vi "Add Alarm_Alarm.vi"(7 "SysDef Ref":T1, 8 "error in (no error)":errorcluster, 9 "Alarm Settings":T2={"Name"="", "Description"="", "Alarm Channel Node Path"="", "UpperLimit"=0.0, "Upper Limit Channel Node Path"="", "LowerLimit"=0.0, "Lower Limit Channel Node Path"="", "Alarm Action Node Path"="", "Mode"=0, "DefaultState"=1, "Priority"=0, "Delay"=0.0, "TripMessage"="", "GroupNumber"=0} {"Priority" items=["Low", "Medium", "High"]; "DefaultState" items=["Disabled", "Enabled"]; "Mode" items=["Normal", "IndicateOnly"]}, 11 "Alarm Folder Ref":refnum<k24>) -> (0 "error out":errorcluster, 3 "Alarm Folder Ref out":refnum<k24>)   [LabVIEW 2019, in "Simple SysDef API.lvlib"]
uses:
  <userlib>/SimpleSysDef/Simple SysDef API.lvlib
  NationalInstruments.VeriStand.SystemDefinitionAPI
  <userlib>/SimpleSysDef/_SubVIs/Add Alarm_Settings.ctl
  <userlib>/SimpleSysDef/_SubVIs/System Definition Reference.ctl
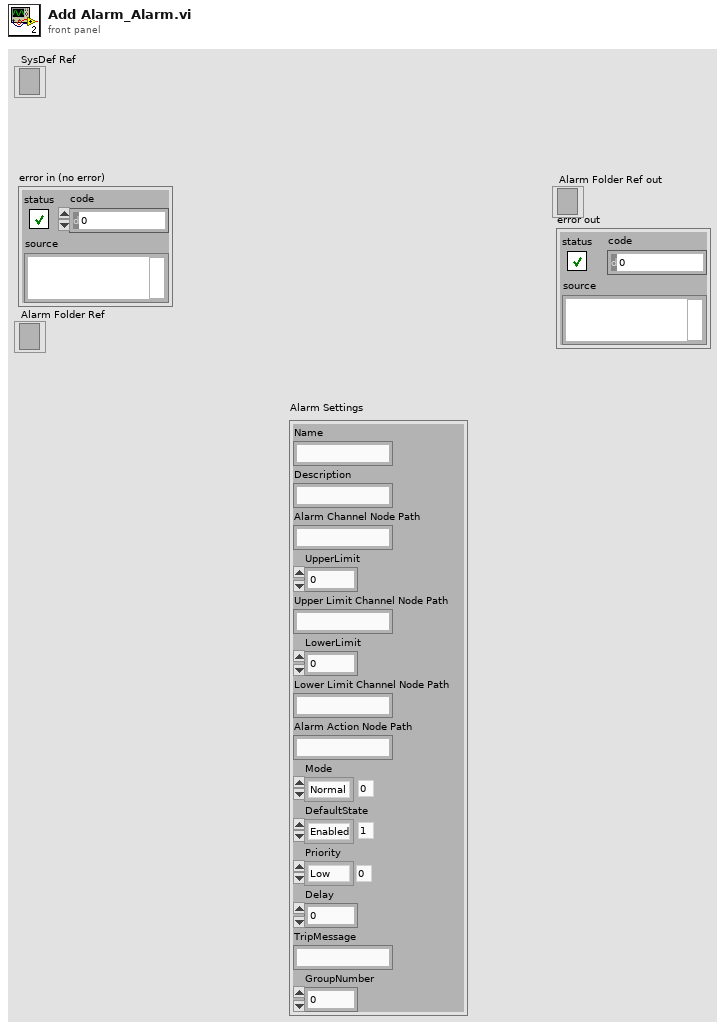
[diagram p1: front panel]
types:
  T1 = typedef "Simple SysDef API.lvlib/System Definition Reference.ctl" = refnum<k24>
  T2 = typedef "Simple SysDef API.lvlib/Add Alarm_Settings.ctl" = cluster{"Name":string, "Description":string, "Alarm Channel Node Path":string, "UpperLimit":dbl, "Upper Limit Channel Node Path":string, "LowerLimit":dbl, "Lower Limit Channel Node Path":string, "Alarm Action Node Path":string, "Mode":i32, "DefaultState":i32, "Priority":i32, "Delay":dbl, "TripMessage":string, "GroupNumber":u32}
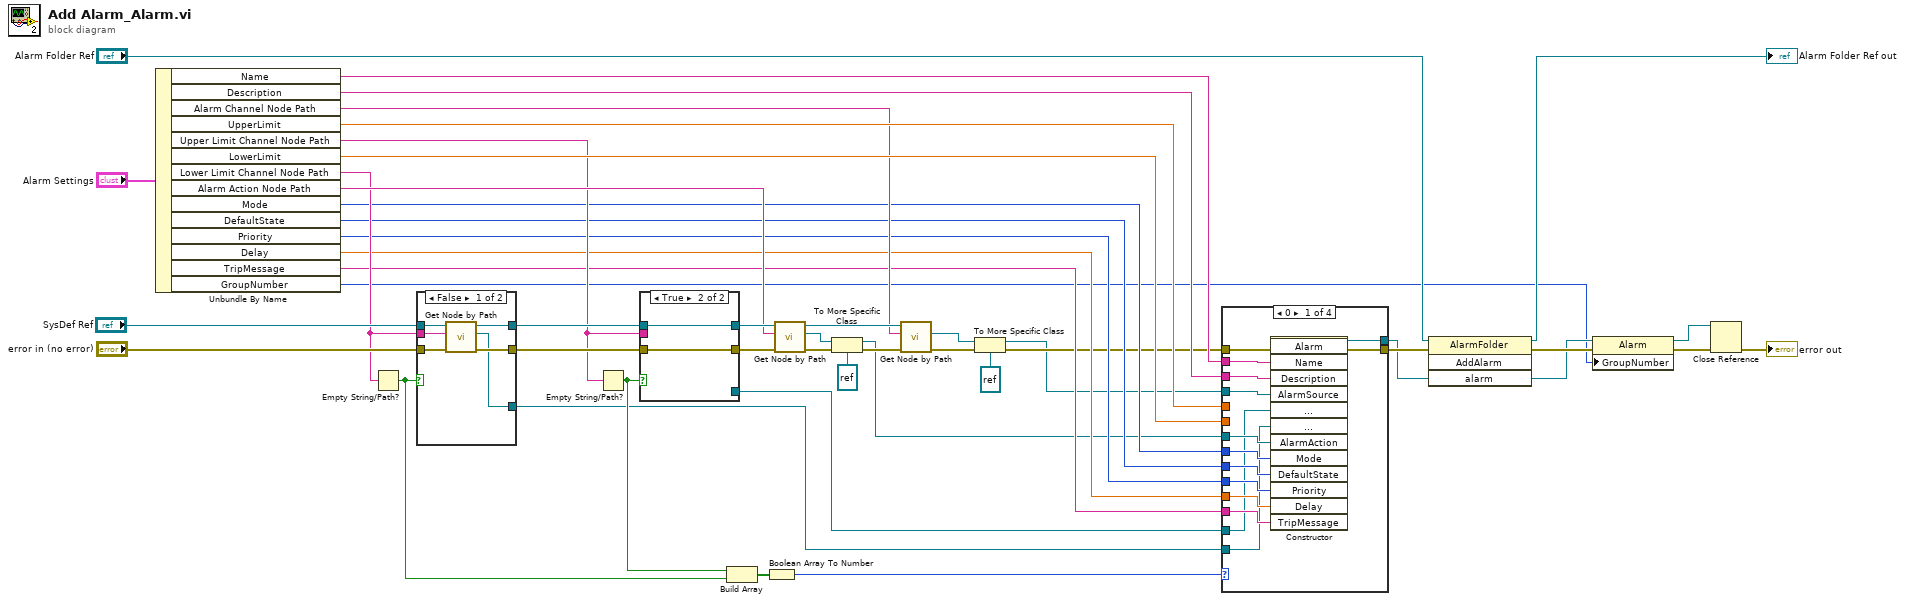
[diagram p0: block diagram]
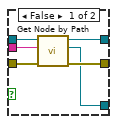
[diagram p2: hidden frame]
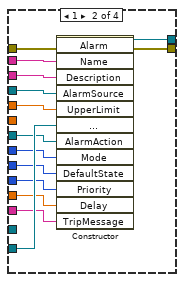
[diagram p4: hidden frame]
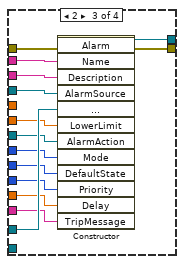
[diagram p5: hidden frame]
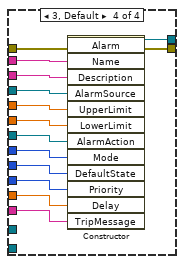
[diagram p6: hidden frame]
diagram:
  n1 = Unbundle By Name("Alarm Settings") -> ("Name"=w25:string, "Description"=w24:string, "Alarm Channel Node Path"=w21:string, "UpperLimit"=w23:dbl, "Upper Limit Channel Node Path"=w19:string, "LowerLimit"=w22:dbl, "Lower Limit Channel Node Path"=w18:string, "Alarm Action Node Path"=w20:string, "Mode"=w17:i32, "DefaultState"=w16:i32, "Priority"=w15:i32, "Delay"=w14:dbl, "TripMessage"=w13:string, "GroupNumber"=w12:u32)
  n2 = Empty String/Path?(string/path=w18) -> (empty?=w35:bool)
  n3 = case shown="False" w35 {
    tunnel: "error in (no error)" -> [w52 w54]
    tunnel: [w51 w54] -> w37
    tunnel: "SysDef Ref" -> [w50 w53]
    tunnel: [w49 w53] -> w38
    tunnel: [w48 _] -> w11
    tunnel: w18 -> [w47 _]
    frame False {
      n4 = call <userlib>:"Get Node by Path.vi"("error in (no error)"=w52, "System Definition Node Path"=w47, "SysDef Ref"=w50) -> ("error out"=w51:errorcluster, "Node Ref"=w48:refnum<k24>, "SysDef Ref Out"=w49:T1)  [unwired: 6 in]
    }
    frame True {
    }
  }
  n5 = Empty String/Path?(string/path=w19) -> (empty?=w36:bool)
  n6 = case shown="True" w36 {
    tunnel: w37 -> [w60 w62]
    tunnel: [w59 w62] -> w33
    tunnel: w38 -> [w58 w61]
    tunnel: [w57 _] -> w10
    tunnel: w19 -> [w56 _]
    tunnel: [w55 w61] -> w30
    frame False {
      n7 = call <userlib>:"Get Node by Path.vi"("error in (no error)"=w60, "System Definition Node Path"=w56, "SysDef Ref"=w58) -> ("error out"=w59:errorcluster, "Node Ref"=w57:refnum<k24>, "SysDef Ref Out"=w55:T1)  [unwired: 6 in]
    }
    frame True {
    }
  }
  n8 = Build Array(w36, w35) -> (w34:bool[])
  n9 = Boolean Array To Number(Boolean array=w34) -> (number=w29:u32)
  n10 = call <userlib>:"Get Node by Path.vi"("error in (no error)"=w33, "System Definition Node Path"=w20, "SysDef Ref"=w30) -> ("error out"=w28:errorcluster, "Node Ref"=w7:refnum<k24>, "SysDef Ref Out"=w27:T1)  [unwired: 6 in]
  n11 = To More Specific Class(target class=refnum<k24> refnum ("AlarmAction"), reference=w7, error in=w28) -> (specific class reference=w6:refnum<k24>, error out=w9:errorcluster)
  n12 = call <userlib>:"Get Node by Path.vi"("error in (no error)"=w9, "System Definition Node Path"=w21, "SysDef Ref"=w27) -> ("error out"=w5:errorcluster, "Node Ref"=w3:refnum<k24>)  [unwired: 6 in, 1 out]
  n13 = To More Specific Class(target class=refnum<k24> refnum ("AlarmSource"), reference=w3, error in=w5) -> (specific class reference=w2:refnum<k24>, error out=w4:errorcluster)
  n14 = case shown="0" w29 {
    tunnel: [w76 w90 w103 w117] -> w45
    tunnel: [w75 w89 w104 w118] -> w43
    tunnel: w4 -> [w74 w88 w102 w116]
    tunnel: w6 -> [w68 w82 w96 w106]
    tunnel: w2 -> [w65 w85 w99 w105]
    tunnel: w25 -> [w63 w87 w101 w115]
    tunnel: w24 -> [w64 w86 w100 w114]
    tunnel: w23 -> [_ w84 _ w113]
    tunnel: w22 -> [_ _ w97 w112]
    tunnel: w17 -> [w69 w81 w95 w111]
    tunnel: w16 -> [w70 w80 w94 w110]
    tunnel: w15 -> [w71 w79 w93 w109]
    tunnel: w14 -> [w72 w78 w92 w108]
    tunnel: w13 -> [w73 w77 w91 w107]
    tunnel: w11 -> [w67 w83 _ _]
    tunnel: w10 -> [w66 _ w98 _]
    frame 0 {
      n15 = constructor class="Alarm"(error in=w74, "Name"=w63, "Description"=w64, "AlarmSource"=w65, "UpperLimit"=w66, "LowerLimit"=w67, "AlarmAction"=w68, "Mode"=w69, "DefaultState"=w70, "Priority"=w71, "Delay"=w72, "TripMessage"=w73) -> (reference out=w75:refnum<k24>, error out=w76:errorcluster)  [unwired: 2 in, 12 out]
    }
    frame 1 {
      n16 = constructor class="Alarm"(error in=w88, "Name"=w87, "Description"=w86, "AlarmSource"=w85, "UpperLimit"=w84, "LowerLimit"=w83, "AlarmAction"=w82, "Mode"=w81, "DefaultState"=w80, "Priority"=w79, "Delay"=w78, "TripMessage"=w77) -> (reference out=w89:refnum<k24>, error out=w90:errorcluster)  [unwired: 2 in, 12 out]
    }
    frame 2 {
      n17 = constructor class="Alarm"(error in=w102, "Name"=w101, "Description"=w100, "AlarmSource"=w99, "UpperLimit"=w98, "LowerLimit"=w97, "AlarmAction"=w96, "Mode"=w95, "DefaultState"=w94, "Priority"=w93, "Delay"=w92, "TripMessage"=w91) -> (reference out=w104:refnum<k24>, error out=w103:errorcluster)  [unwired: 2 in, 12 out]
    }
    frame 3, Default {
      n18 = constructor class="Alarm"(error in=w116, "Name"=w115, "Description"=w114, "AlarmSource"=w105, "UpperLimit"=w113, "LowerLimit"=w112, "AlarmAction"=w106, "Mode"=w111, "DefaultState"=w110, "Priority"=w109, "Delay"=w108, "TripMessage"=w107) -> (reference out=w118:refnum<k24>, error out=w117:errorcluster)  [unwired: 2 in, 12 out]
    }
  }
  n19 = invoke class="AlarmFolder" method="AddAlarm"(reference="Alarm Folder Ref", error in=w45, "alarm"=w43) -> (reference out=→"Alarm Folder Ref out":refnum<k24>, error out=w44:errorcluster)  [unwired: 1 in, 2 out]
  n20 = property class="Alarm"(reference=w43, error in=w44, "GroupNumber"=w12) -> (reference out=w42:refnum<k24>, error out=w41:errorcluster)
  n21 = Close Reference(reference=w42, error in (no error)=w41) -> (error out=→"error out":errorcluster)
